vi "Test_Final.vi"() -> ()   [LabVIEW 2015]
uses:
  <vilib>/ErrorRing/Error Ring.xnode
panel:
  in  "Instructions":bool
  out "Test":string
  out "Index_Display":i32
  out "Score":i32
  in  "Start Button":bool
  in  "Boolean 4":bool
  in  "Boolean 3":bool
  in  "Boolean 2":bool
  in  "Boolean":bool
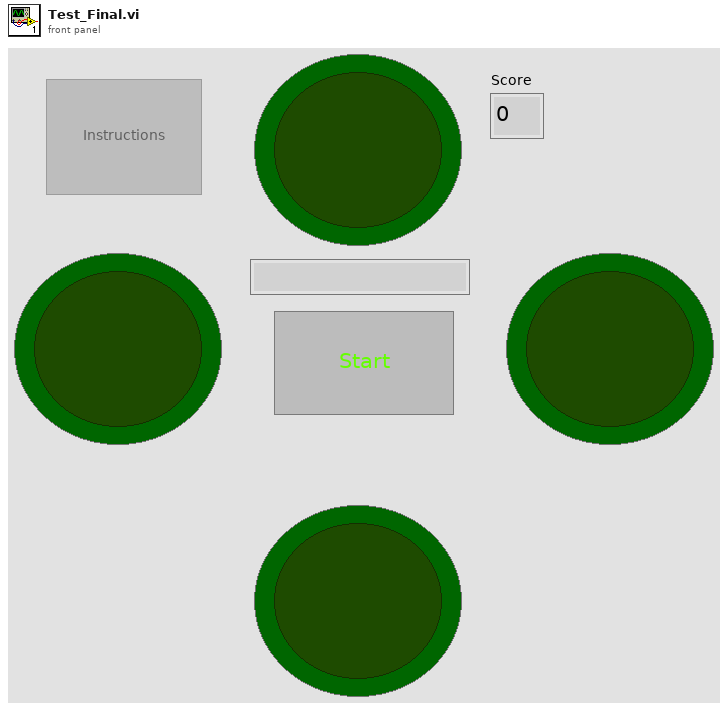
[diagram p1: front panel]
types:
  T1 = enum8{"Enabled", "Disabled", "Disabled and Grayed Out"}
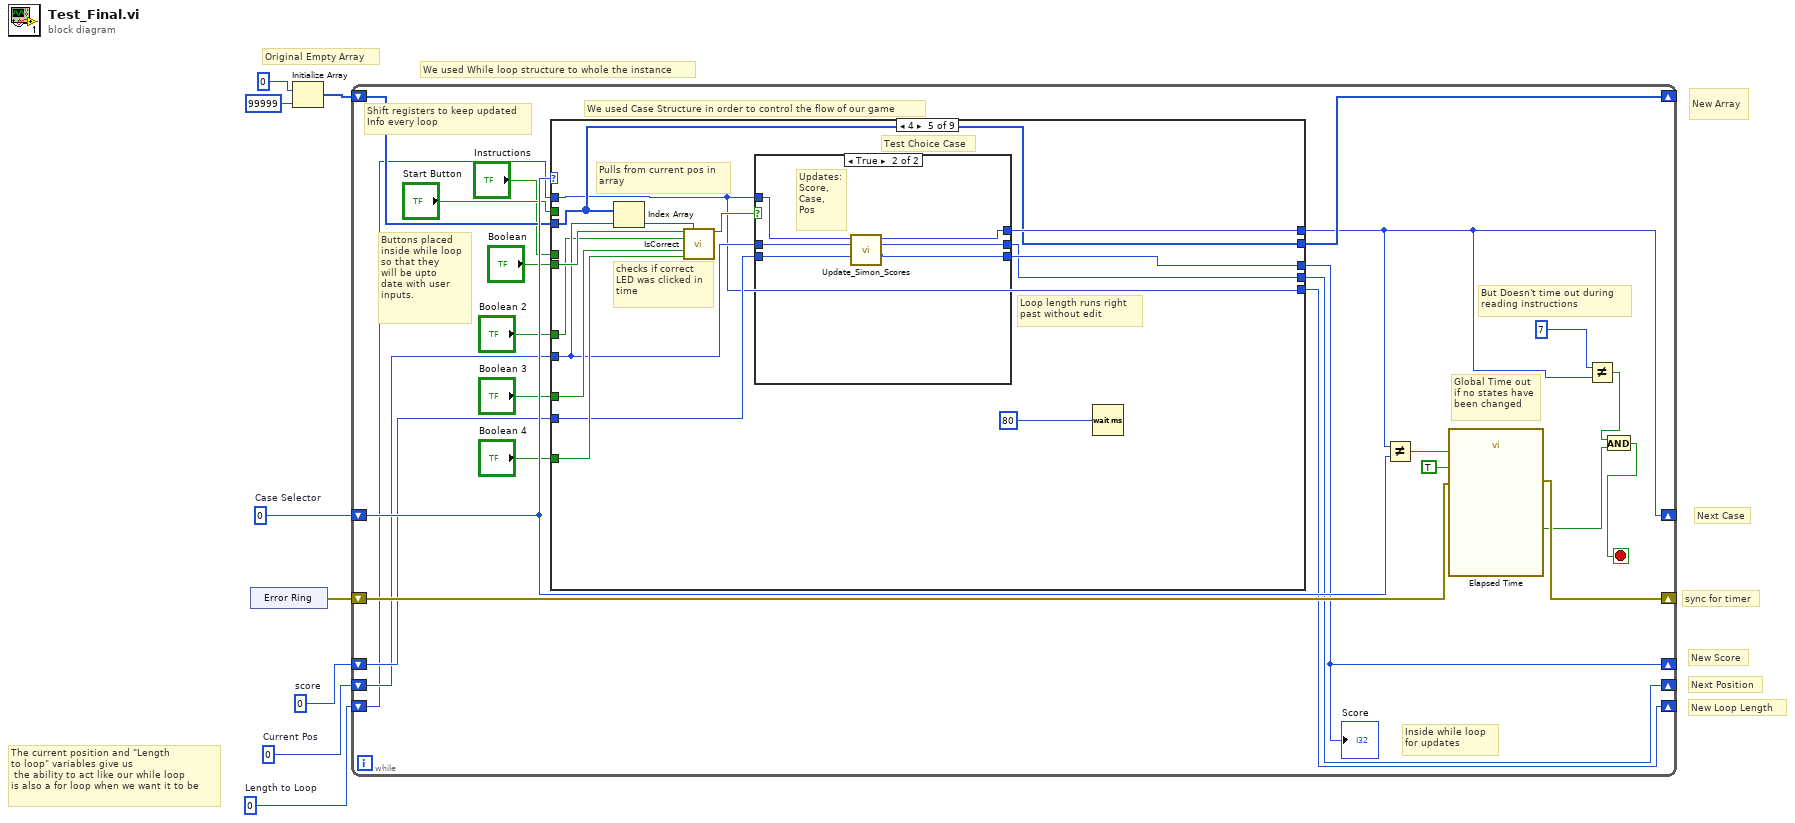
[diagram p0: block diagram]
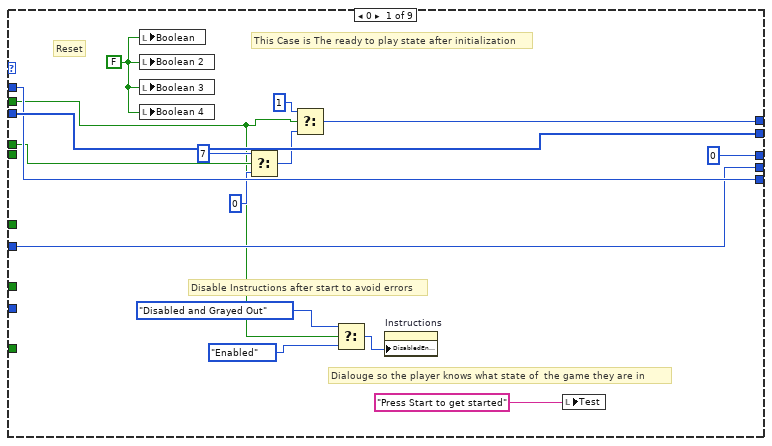
[diagram p2: hidden frame]
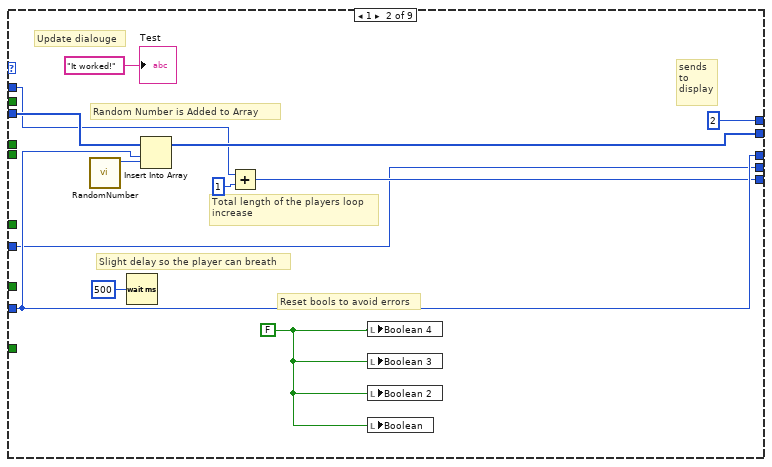
[diagram p3: hidden frame]
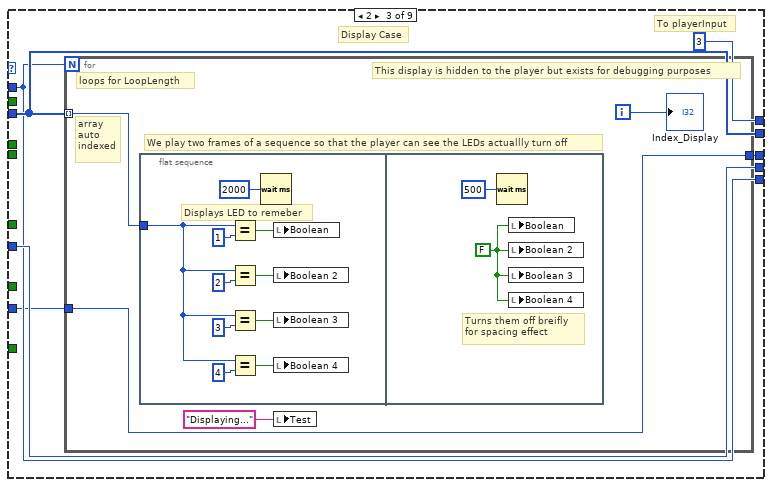
[diagram p4: hidden frame]
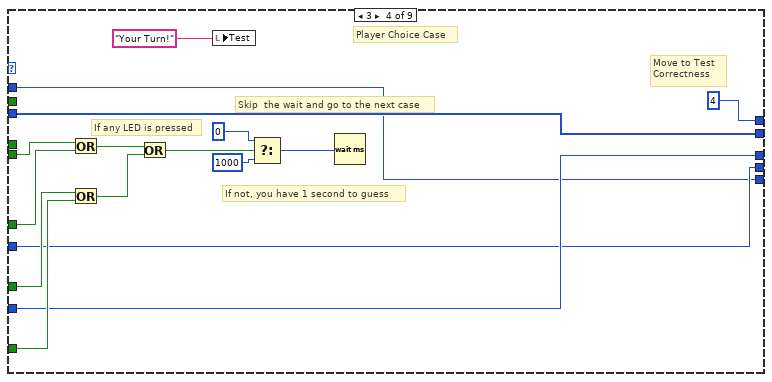
[diagram p5: hidden frame]
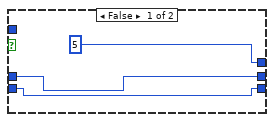
[diagram p6: hidden frame]
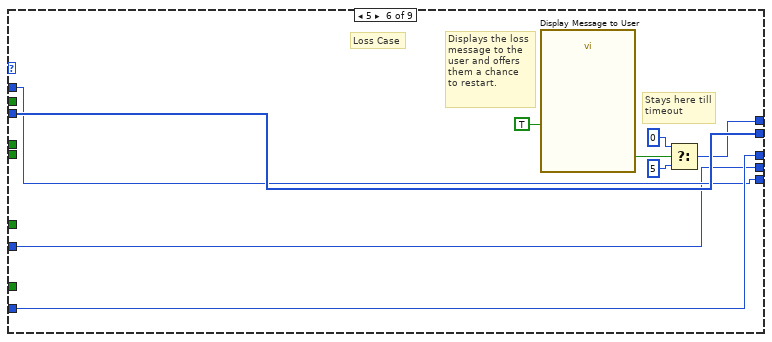
[diagram p7: hidden frame]
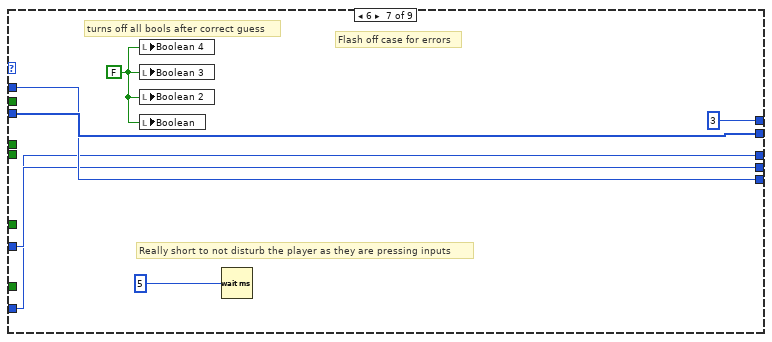
[diagram p8: hidden frame]
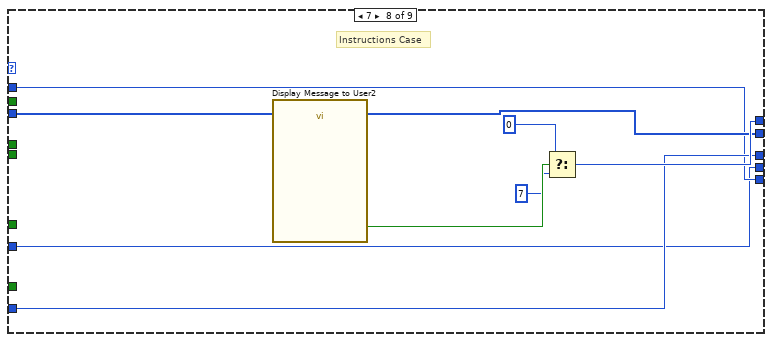
[diagram p9: hidden frame]
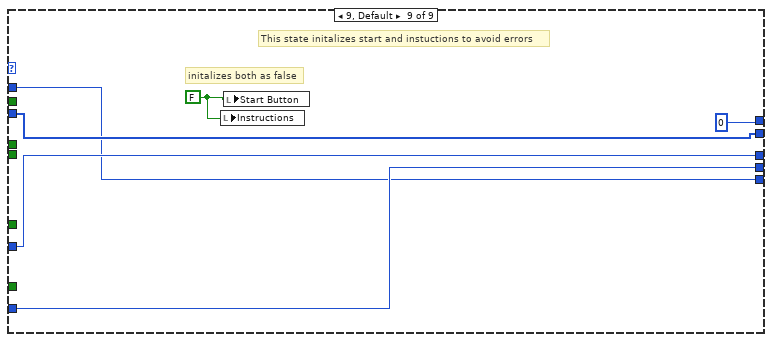
[diagram p10: hidden frame]
diagram:
  w2 = 0  # Length to Loop
  w3 = 0  # Current Pos
  w7 = 0  # score
  w8 = 0  # Case Selector
  # "We used While loop structure to whole the instance"
  # "sync for timer"
  # "New Loop Length"
  # "Next Position"
  # "New Score"
  # "Next Case"
  # "New Array"
  # "The current position and \"Length \nto loop\" variables give us\n the ability to act like our while loop\nis also a for loop when we want it to be"
  # "Original Empty Array"
  n1 = xnode "Error Ring"() -> ("error out"=w1:errorcluster)
  n2 = Initialize Array(0 ("element"), 99999 ("dimension size")) -> (w4:i32[])
  n3 = while {
    shift-right: [w30] -> _
    shift-left: w1 -> [w29]
    shift-right: [w12] -> _
    shift-left: w8 -> [w28]
    shift-right: [w24] -> _
    shift-left: w7 -> [w26]
    shift-right: [w25] -> _
    shift-left: w4 -> [w27]
    shift-right: [w21] -> _
    shift-left: w2 -> [w22]
    shift-right: [w20] -> _
    shift-left: w3 -> [w23]
    stop <- w9 stop-if-true
    # "We used Case Structure in order to control the flow of our game"
    # "But Doesn't time out during\nreading instructions"
    # "Global Time out\nif no states have\nbeen changed"
    # "Inside while loop \nfor updates"
    # "Buttons placed\ninside while loop\nso that they \nwill be upto\ndate with user\ninputs."
    # "Shift registers to keep updated \nInfo every loop"
    n4 = case shown="4" w28 {
      tunnel: "Start Button" -> [w36 _ _ _ _ _ _ _ _]
      tunnel: [w47 2 ("f") 3 ("f") 4 ("f") w106 w125 3 ("f") w142 0 ("f")] -> w12
      tunnel: w27 -> [w45 w59 w66 w87 w104 w130 w136 w140 w150]
      tunnel: w26 -> [_ w55 w61 w86 w108 w124 w133 w141 w148]
      tunnel: [w45 w58 w66 w87 w104 w130 w136 w140 w150] -> w25
      tunnel: [0 ("score") w55 w62 w86 w107 w124 w133 w141 w149] -> w24
      tunnel: "Boolean" -> [_ _ _ w96 w112 _ _ _ _]
      tunnel: "Boolean 2" -> [_ _ _ w95 w99 _ _ _ _]
      tunnel: "Boolean 3" -> [_ _ _ w94 w111 _ _ _ _]
      tunnel: "Boolean 4" -> [_ _ _ w93 w110 _ _ _ _]
      tunnel: w23 -> [w43 w51 w65 w85 w103 w122 w134 w138 w149]
      tunnel: w22 -> [w44 w54 w63 w84 w101 w123 w135 w139 w147]
      tunnel: [w44 w52 w63 w84 w101 w123 w135 w139 w147] -> w21
      tunnel: [w43 w51 w65 w85 w102 w122 w134 w138 w148] -> w20
      tunnel: "Instructions" -> [w40 _ _ _ _ _ _ _ _]
      frame 0 {
        w42 = FALSE ("Boolean")
        # "Disable Instructions after start to avoid errors"
        # "Dialouge so the player knows what state of  the game they are in"
        # "This Case is The ready to play state after initialization"
        # "Reset"
        n5 = local write "Boolean"(w42) -> ()
        n6 = local write "Boolean 2"(w42) -> ()
        n7 = local write "Boolean 3"(w42) -> ()
        n8 = local write "Boolean 4"(w42) -> ()
        n9 = Select(t=7, s=w40, f=0 ("t")) -> (s? t:f=w38:i32)
        n10 = Select(t=1, s=w36, f=w38) -> (s? t:f=w47:i32)
        n11 = Select(t=T1."Disabled and Grayed Out" ("Disabled"), s=w36, f=T1."Enabled" ("Disabled")) -> (s? t:f=w33:T1)
        n12 = property on="Instructions" class="Bool (strict)"("DisabledEnum"=w33) -> ()  [unwired: 2 in, 2 out]
        n13 = local write "Test"("Press Start to get started" ("Test")) -> ()
      }
      frame 1 {
        w49 = FALSE ("Boolean 4")
        # "sends\nto\ndisplay"
        # "Reset bools to avoid errors"
        # "Slight delay so the player can breath"
        # "Total length of the players loop\nincrease"
        # "Random Number is Added to Array"
        # "Update dialouge"
        n14 = call "RandomNumber.vi"() -> ("Numeric"=w57:i32)  [unwired: 11 in]
        n15 = Wait (ms)(milliseconds to wait=u32 500) -> ()  [unwired: 1 out]
        n16 = Insert Into Array(array=w59, index=w55, new element=w57) -> (w58:i32[])
        n17 = Add(x=w54, y=1) -> (x+y=w52:i32)
        n18 = local write "Boolean 4"(w49) -> ()
        n19 = local write "Boolean 3"(w49) -> ()
        n20 = local write "Boolean 2"(w49) -> ()
        n21 = local write "Boolean"(w49) -> ()
        "Test" <- "It worked!"
      }
      frame 2 {
        # "Display Case"
        # "To playerInput"
        n22 = for {
          N: w63 -> [_]
          tunnel: w66 -> [w69] mode=indexing
          tunnel: w61 -> [w68]
          tunnel: [w68] -> w62
          i -> [w70]
          # "array\nauto\nindexed"
          # "loops for LoopLength"
          # "We play two frames of a sequence so that the player can see the LEDs actuallly turn off"
          # "This display is hidden to the player but exists for debugging purposes"
          n23 = flat-sequence {
            tunnel: w69 -> [w74]
            frame #0 {
              # "Displays LED to remeber"
              n24 = Equal?(x=w74, y=1) -> (x = y?=w80:bool)
              n25 = Equal?(x=w74, y=2) -> (x = y?=w77:bool)
              n26 = Equal?(x=w74, y=3) -> (x = y?=w78:bool)
              n27 = Equal?(x=w74, y=4) -> (x = y?=w79:bool)
              n28 = Wait (ms)(milliseconds to wait=u32 2000) -> ()  [unwired: 1 out]
              n29 = local write "Boolean"(w80) -> ()
              n30 = local write "Boolean 2"(w77) -> ()
              n31 = local write "Boolean 3"(w78) -> ()
              n32 = local write "Boolean 4"(w79) -> ()
            }
            frame #1 {
              w82 = FALSE ("Boolean 4")
              # "Turns them off breifly \nfor spacing effect"
              n33 = Wait (ms)(milliseconds to wait=u32 500 ("x")) -> ()  [unwired: 1 out]
              n34 = local write "Boolean"(w82) -> ()
              n35 = local write "Boolean 2"(w82) -> ()
              n36 = local write "Boolean 3"(w82) -> ()
              n37 = local write "Boolean 4"(w82) -> ()
            }
          }
          n38 = local write "Test"("Displaying..." ("Test")) -> ()
          "Index_Display" <- w70
        }
      }
      frame 3 {
        # "Move to Test \nCorrectness"
        # "Player Choice Case"
        # "If not, you have 1 second to guess"
        # "Skip  the wait and go to the next case"
        # "If any LED is pressed"
        n39 = Or(x=w96, y=w95) -> (x .or. y?=w98:bool)
        n40 = Or(x=w94, y=w93) -> (x .or. y?=w97:bool)
        n41 = Or(x=w98, y=w97) -> (x .or. y?=w92:bool)
        n42 = local write "Test"("Your Turn!" ("Test")) -> ()
        n43 = Select(t=u32 0 ("milliseconds to wait"), s=w92, f=u32 1000 ("milliseconds to wait")) -> (s? t:f=w89:u32)
        n44 = Wait (ms)(milliseconds to wait=w89) -> ()  [unwired: 1 out]
      }
      frame 4 {
        # "Test Choice Case"
        # "Pulls from current pos in\narray"
        # "Loop length runs right \npast without edit"
        # "checks if correct\nLED was clicked in\ntime"
        n45 = Index Array(array=w104, index=w103) -> (element=w109:i32)
        n46 = call "IsCorrect.vi"("Boolean"=w112, "InValue"=w109, "Boolean 2"=w99, "Boolean 3"=w111, "Boolean 4"=w110) -> ("IsCorrect"=w105:bool)  [unwired: 10 in]
        n47 = case shown="True" w105 {
          tunnel: [5 ("f") w117] -> w106
          tunnel: w108 -> [w114 w119]
          tunnel: [w114 w118] -> w107
          tunnel: w103 -> [w113 w120]
          tunnel: [w113 w116] -> w102
          tunnel: w101 -> [_ w121]
          frame False {
          }
          frame True {
            # "Updates:\nScore,\nCase,\nPos"
            n48 = call "Update_Simon_Scores.vi"("Score"=w119, "Position"=w120, "LoopLength"=w121) -> ("New Score"=w118:i32, "Next Pos"=w116:i32, "Case Selector"=w117:i32)  [unwired: 6 in]
          }
        }
        n49 = Wait (ms)(milliseconds to wait=u32 80) -> ()  [unwired: 1 out]
      }
      frame 5 {
        # "Loss Case"
        # "Stays here till\ntimeout"
        # "Displays the loss\nmessage to the \nuser and offers\nthem a chance \nto restart."
        n50 = call "Display Message to User"("Enable"=TRUE) -> ("OK"=w128:bool)  [unwired: 9 in, 1 out]
        n51 = Select(t=0, s=w128, f=5) -> (s? t:f=w125:i32)
      }
      frame 6 {
        w132 = FALSE ("Boolean 4")
        # "turns off all bools after correct guess"
        # "Really short to not disturb the player as they are pressing inputs"
        # "Flash off case for errors"
        n52 = local write "Boolean 4"(w132) -> ()
        n53 = local write "Boolean 3"(w132) -> ()
        n54 = local write "Boolean 2"(w132) -> ()
        n55 = local write "Boolean"(w132) -> ()
        n56 = Wait (ms)(milliseconds to wait=u32 5) -> ()  [unwired: 1 out]
      }
      frame 7 {
        # "Instructions Case"
        n57 = call "Display Message to User2"() -> ("OK"=w145:bool)  [unwired: 10 in, 1 out]
        n58 = Select(t=0 ("f"), s=w145, f=7) -> (s? t:f=w142:i32)
      }
      frame 9, Default {
        w146 = FALSE ("Start Button")
        # "initalizes both as false"
        # "This state initalizes start and instuctions to avoid errors"
        n59 = local write "Instructions"(w146) -> ()
        n60 = local write "Start Button"(w146) -> ()
      }
    }
    "Score" <- w24
    n61 = Not Equal?(x=w12, y=w28) -> (x != y?=w31:bool)
    n62 = call "Elapsed Time"("Reset"=w31, "Auto Reset"=TRUE, "error in (no error)"=w29) -> ("Time has Elapsed"=w10:bool, "error out"=w30:errorcluster)  [unwired: 9 in, 6 out]
    n63 = Not Equal?(x=7 ("t"), y=w12) -> (x != y?=w11:bool)
    n64 = And(x=w11, y=w10) -> (x .and. y?=w9:bool)
  }
